vi "保存数据.vi"(6 "备注":string="111", 7 "状态数据":string[](array[string])=["关", "正常", "1000000", "1055.98389", "NaN", "43601.9()", "43601.9()", "Inf", "0.01611", "11.4", "0.7()", "0.7()", "0.0", "0.00916", "4.99969", "1.16279", "0.08759"], 8 "应用程序输入":refnum<vi>, 9 "SN":string="8716445348498350066CFF55", 11 "型号":string) -> ()   [LabVIEW 2015]
uses:
  <vilib>/addons/_office/_exclsub.llb/font.ctl
  Globle.vi
  <vilib>/addons/_office/excel.llb/Excel Get Data (str).vi
  <vilib>/addons/_office/excel.llb/Excel Easy Table (str).vi
  <vilib>/Utility/NIReport.llb/NI_report.lvclass
  <vilib>/addons/_office/NI_ReportGenerationToolkit.lvlib
  <vilib>/Utility/NIReport.llb/Excel/NI_Excel.lvclass
panel:
  out "写入行位置":i32
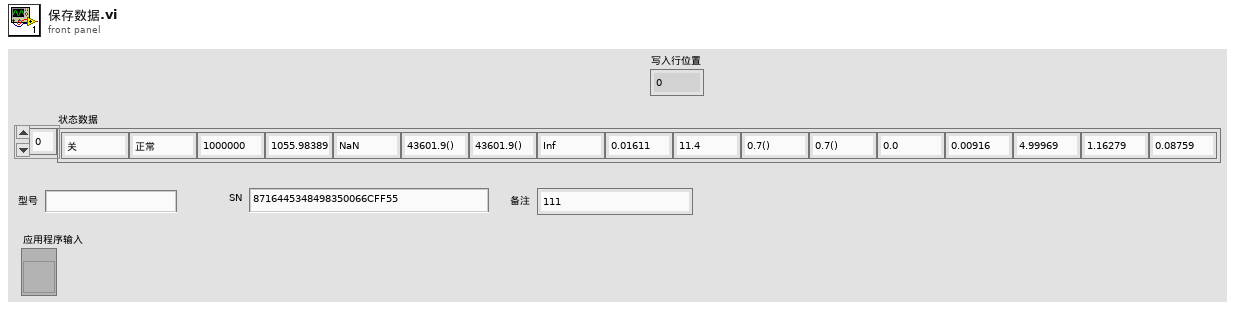
[diagram p1: front panel]
types:
  T1 = enum16{"maximized", "minimized", "normal", "no change"}
  T2 = enum16{"Standard Report", "HTML", "Word", "Excel"}
  T3 = typedef "NI_ReportGenerationToolkit.lvlib/font.ctl" = cluster{"font name":string, "font size":dbl, "bold":u16, "italic":u16, "underline":u16, "strike through":u16, "font color":u32}
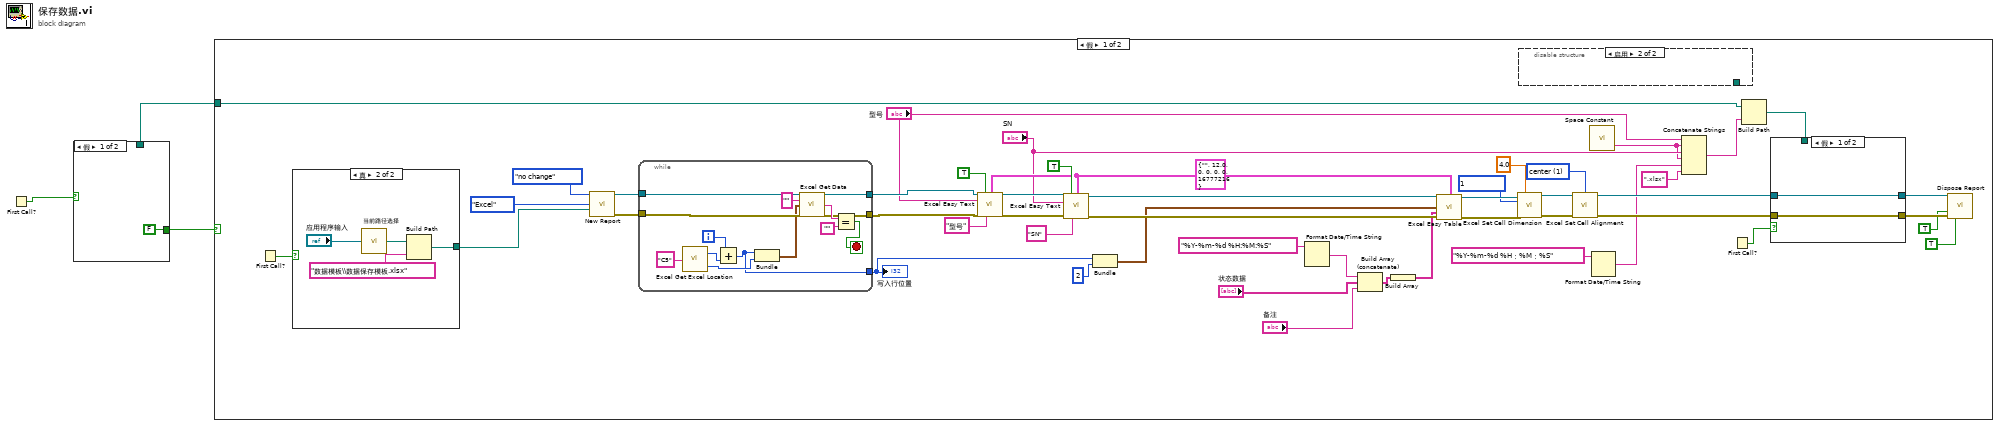
[diagram p0: block diagram]
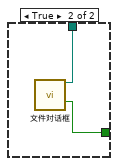
[diagram p2: hidden frame]
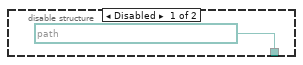
[diagram p3: hidden frame]
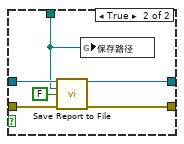
[diagram p4: hidden frame]
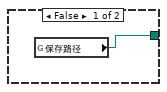
[diagram p5: hidden frame]
diagram:
  n1 = First Call?() -> (First Call?: T/F=w2:bool)
  n2 = case shown="假" w2 {
    tunnel: [FALSE ("cancelled") w6] -> w3
    tunnel: [_ w5] -> w1
    frame False {
    }
    frame True {
      n3 = call "文件对话框"() -> ("selected path"=w5:path, "cancelled"=w6:bool)  [unwired: 12 in, 2 out]
    }
  }
  n4 = case shown="假" w3 {
    tunnel: w1 -> [w7 _]
    frame False {
      w25 = 1 items=["left", "center", "right"] ("horizontal alignment (left)")
      w28 = T3 {"font name"="", "font size"=12.0, "bold"=0, "italic"=0, "underline"=0, "strike through"=0, "font color"=16777216} ("font")
      n5 = First Call?() -> (First Call?: T/F=w9:bool)
      n6 = case shown="真" w9 {
        tunnel: [w65 w66] -> w55
        frame False {
          n7 = global read "Globle.vi" "保存路径"() -> (w65:path)
        }
        frame True {
          n8 = call "当前路径选择.vi"("本应用程序"="应用程序输入") -> ("当前路径"=w68:path)
          n9 = Build Path(base path=w68, name or relative path="数据模板\\数据保存模板.xlsx" ("名称或相对路径")) -> (appended path=w66:path)
        }
      }
      n10 = call <vilib>:"New Report.vi"("window state (normal)"=T1."no change", "report type"=T2."Excel", "template (empty)"=w55) -> ("report out"=w52:refnum<class "NI_report.lvclass">, "error out"=w51:errorcluster)  [unwired: 11 in]
      n11 = while {
        tunnel: w52 -> [w83]
        tunnel: w51 -> [w82]
        tunnel: [w73] -> w50
        tunnel: [w71] -> w47
        tunnel: [w70] -> w46
        i -> [w80]
        stop <- w74 stop-if-true
        n12 = call <vilib>:"Excel Get Excel Location.vi"("cell's name"="C5") -> ("row"=w79:i32, "column"=w78:i32)
        n13 = Add(x=w80, y=w79) -> (x+y=w73:i32)
        n14 = Bundle(w73, "column"=w78) -> (w77:cluster{i32, "column":i32})  [unwired: 1 in]
        n15 = call-poly <vilib>:"Excel Get Data.vi"("report in"=w83, "data type"="", "start (0, 0)"=w77, "error in (no error)"=w82) -> ("report out"=w71:refnum<class "NI_report.lvclass">, "data"=w76:string, "error out"=w70:errorcluster)  [unwired: 9 in]
        n16 = Equal?(x=w76, y="") -> (x = y?=w74:bool)
      }
      "写入行位置" <- w50
      n17 = call <vilib>:"Excel Easy Text.vi"("report in"=w47, "border? (F)"=TRUE, "font"=w28, "text"="型号", "error in (no error)"=w46, "name (\"\")"="型号" ("name (\"\")")) -> ("report out"=w45:refnum<class "NI_report.lvclass">, "error out"=w44:errorcluster)  [unwired: 5 in, 3 out]
      n18 = call <vilib>:"Excel Easy Text.vi"("report in"=w45, "border? (F)"=TRUE, "font"=w28, "text"="SN", "error in (no error)"=w44, "name (\"\")"="SN" ("name (\"\")")) -> ("report out"=w43:refnum<class "NI_report.lvclass">, "error out"=w42:errorcluster)  [unwired: 5 in, 3 out]
      n19 = Bundle(w50, 2) -> (w31:cluster{i32, i32})  [unwired: 1 in]
      n20 = Format Date/Time String(time format string (%c)="%Y-%m-%d %H:%M:%S" ("时间格式字符串(%c)")) -> (date/time string=w20:string)  [unwired: 2 in]
      n21 = Build Array (concatenate)(w20, "状态数据", "备注") -> (w38:string[])
      n22 = Build Array(w38) -> (w37:string[][])
      n23 = call-poly <vilib>:"Excel Easy Table.vi"("report in"=w43, "font"=w28, "start (0, 0)"=w31, "text data"=w37, "error in (no error)"=w42) -> ("report out"=w34:refnum<class "NI_report.lvclass">, "error out"=w35:errorcluster)  [unwired: 6 in, 3 out]
      n24 = call <vilib>:"Excel Set Cell Dimension.vi"("report in"=w34, "width (-1)"=4.0, "measurement system"=u16 1, "error in (no error)"=w35) -> ("report out"=w26:refnum<class "NI_report.lvclass">, "error out"=w27:errorcluster)  [unwired: 10 in]
      n25 = disable-structure shown="启用" {
        disable-tunnel: [path "D:/项目/MPZ2006固态源/数据保存" ("路径") _] -> _
        frame Disabled {
        }
        frame Enabled {
        }
      }
      n26 = call <vilib>:"Excel Set Cell Alignment.vi"("report in"=w26, "horizontal alignment (left)"=w25, "error in (no error)"=w27) -> ("report out"=w23:refnum<class "NI_report.lvclass">, "error out"=w24:errorcluster)  [unwired: 11 in]
      n27 = call <vilib>:"Space Constant.vi"() -> ("String"=w14:string)
      n28 = Format Date/Time String(time format string (%c)="%Y-%m-%d %H：%M：%S" ("时间格式字符串(%c)")) -> (date/time string=w11:string)  [unwired: 2 in]
      n29 = Concatenate Strings("型号", w14, "SN", w14, w11, ".xlsx" ("字符串")) -> (w13:string)
      n30 = First Call?() -> (First Call?: T/F=w8:bool)
      n31 = Build Path(base path=w7, name or relative path=w13) -> (appended path=w10:path)
      n32 = case shown="假" w8 {
        tunnel: w24 -> [w57 w64]
        tunnel: w23 -> [w58 w63]
        tunnel: [w58 w62] -> w18
        tunnel: [w57 w61] -> w17
        tunnel: w10 -> [_ w59]
        frame False {
        }
        frame True {
          n33 = call-dynamic "Save Report to File.vi"("report in"=w63, "report file path"=w59, "prompt to replace? (F)"=FALSE, "error in (no error)"=w64) -> ("report out"=w62:refnum<class "NI_report.lvclass">, "error out"=w61:errorcluster)  [unwired: 10 in]
          n34 = global write "Globle.vi" "保存路径"(w59) -> ()
        }
      }
      n35 = call-dynamic "Dispose Report.vi"("report in"=w18, "save changes? (F)"=TRUE, "error in (no error)"=w17, "close report? (T)"=TRUE) -> ()  [unwired: 11 in, 1 out]
    }
    frame True {
    }
  }
